vi "BK Precision 91xx (GPIB) Initialization VI.vi"(8 "error in (no error)":errorcluster, 10 "Custom XML":string, 11 "Device Item Ref in":T3 format="%.0x") -> (0 "error out":errorcluster, 3 "Device Item Ref out":T3 format="%.0x")   [LabVIEW 2009, in "BK Precision 91xx (GPIB) Custom Device.lvlib"]
uses:
  BK Precision 91xx (GPIB) Custom Device.lvlib
  <vilib>/NI VeriStand/Custom Device API/Custom Device Item Ref.ctl
  <vilib>/NI VeriStand/Custom Device API/Custom Device Channel.ctl
  <vilib>/NI VeriStand/Custom Device API/Custom Device Channel Type.ctl
  <vilib>/NI VeriStand/Custom Device API/Custom Device Timed Loop Priority.ctl
  <vilib>/NI VeriStand/Custom Device API/Custom Device Loop Type.ctl
  <vilib>/NI VeriStand/Custom Device API/Custom Device API.lvlib
panel:
  in  "Enable Channel":T1={"Type"=enum."Input", "Units"="", "Default Value"=0.0, "Faultable"=TRUE, "Scalable"=FALSE}
  in  "Output Channels":T1={"Type"=enum."Output", "Units"="", "Default Value"=0.0, "Faultable"=FALSE, "Scalable"=FALSE}
  in  "Input Channels":T1={"Type"=enum."Input", "Units"="Amps", "Default Value"=0.0, "Faultable"=TRUE, "Scalable"=TRUE}
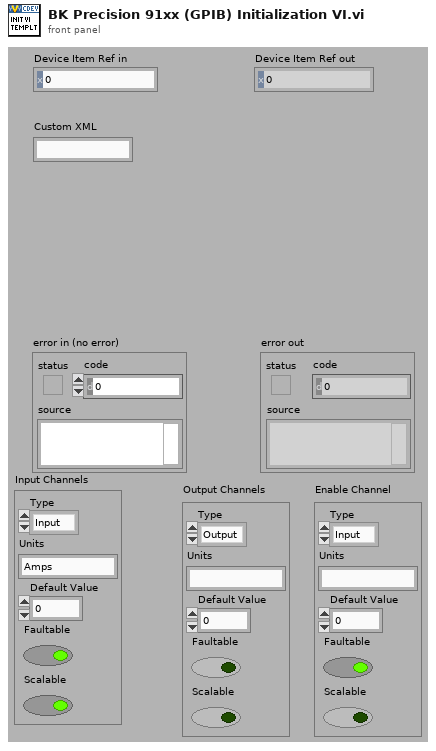
[diagram p1: front panel]
types:
  T1 = typedef "Custom Device API.lvlib/Custom Device Channel.ctl" = cluster{"Type":T2, "Units":string, "Default Value":dbl, "Faultable":bool, "Scalable":bool}
  T2 = typedef "Custom Device API.lvlib/Custom Device Channel Type.ctl" = enum16{"Input", "Output"}
  T3 = typedef "Custom Device API.lvlib/Custom Device Item Ref.ctl" = u64
  T4 = typedef "Custom Device API.lvlib/Custom Device Timed Loop Priority.ctl" = enum32{"Low", "Medium", "High"}
  T5 = typedef "Custom Device API.lvlib/Custom Device Loop Type.ctl" = enum32{"While Loop", "Timed Loop"}
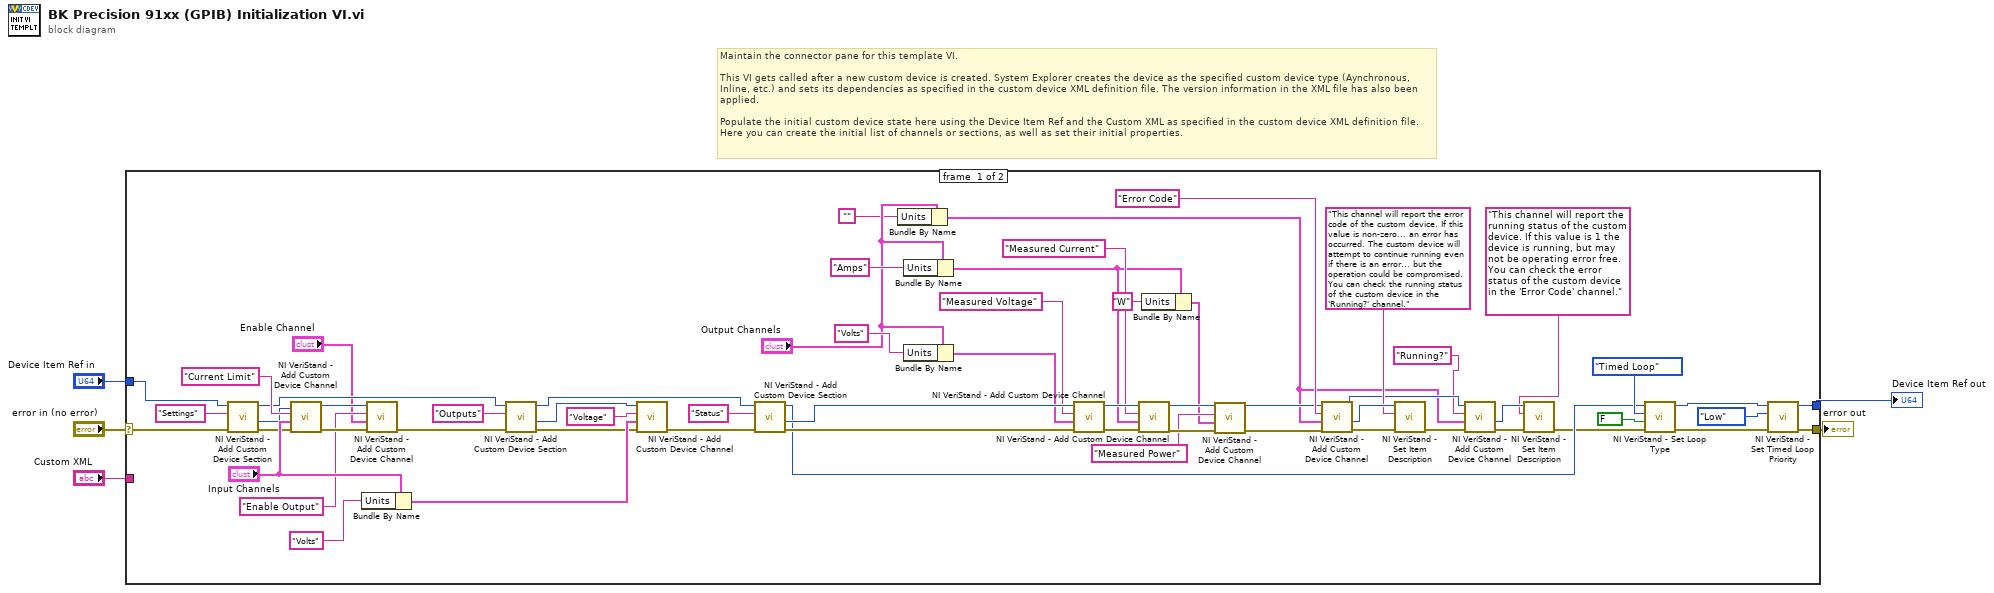
[diagram p0: block diagram]
diagram:
  # "Maintain the connector pane for this template VI.\n\nThis VI gets called after a new custom device is created. System Explorer creates the device as the specified custom device type (Aynchronous, Inline, etc.) and sets its dependencies as specified in the custom device XML definition file. The version information in the XML file has also been applied.\n\nPopulate the initial custom device state here using the Device Item Ref and the Custom XML as specified in the custom device XML definition file. Here you can create the initial list of channels or sections, as well as set their initial properties."
  n1 = case shown="No Error" "error in (no error)" {
    selector: "error in (no error)" -> [w40 w68]
    tunnel: [w48 w68] -> w5
    tunnel: [w45 w67] -> w3
    tunnel: "Device Item Ref in" -> [w41 w67]
    tunnel: "Custom XML" -> [_ _]
    frame #0 {
      n2 = call <vilib>:"NI VeriStand - Add Custom Device Section.vi"("error in (no error)"=w40, "Section Name"="Settings", "Parent Ref in"=w41) -> ("error out"=w36:errorcluster, "Section Ptr"=w39:T3, "Parent Ref out"=w32:T3)  [unwired: 6 in]
      n3 = call <vilib>:"NI VeriStand - Add Custom Device Channel.vi"("error in (no error)"=w36, "Channel"="Input Channels", "Channel Name"="Current Limit", "Parent Ref in"=w39) -> ("error out"=w33:errorcluster, "Parent Ref out"=w31:T3)  [unwired: 5 in, 1 out]
      n4 = Bundle By Name(cluster="Input Channels", "Units"="Volts") -> (w58:T1)
      n5 = call <vilib>:"NI VeriStand - Add Custom Device Channel.vi"("error in (no error)"=w33, "Channel"="Enable Channel", "Channel Name"="Enable Output", "Parent Ref in"=w31) -> ("error out"=w34:errorcluster)  [unwired: 5 in, 2 out]
      n6 = call <vilib>:"NI VeriStand - Add Custom Device Section.vi"("error in (no error)"=w34, "Section Name"="Outputs", "Parent Ref in"=w32) -> ("error out"=w35:errorcluster, "Section Ptr"=w38:T3, "Parent Ref out"=w62:T3)  [unwired: 6 in]
      n7 = call <vilib>:"NI VeriStand - Add Custom Device Channel.vi"("error in (no error)"=w35, "Channel"=w58, "Channel Name"="Voltage", "Parent Ref in"=w38) -> ("error out"=w63:errorcluster)  [unwired: 5 in, 2 out]
      n8 = call <vilib>:"NI VeriStand - Add Custom Device Section.vi"("error in (no error)"=w63, "Section Name"="Status", "Parent Ref in"=w62) -> ("error out"=w57:errorcluster, "Section Ptr"=w56:T3, "Parent Ref out"=w22:T3)  [unwired: 6 in]
      n9 = Bundle By Name(cluster="Output Channels", "Units"="") -> (w7:T1)
      n10 = Bundle By Name(cluster="Output Channels", "Units"="Amps") -> (w18:T1)
      n11 = Bundle By Name(cluster="Output Channels", "Units"="Volts") -> (w50:T1)
      n12 = call <vilib>:"NI VeriStand - Add Custom Device Channel.vi"("error in (no error)"=w57, "Channel"=w50, "Channel Name"="Measured Voltage", "Parent Ref in"=w56) -> ("error out"=w53:errorcluster, "Parent Ref out"=w54:T3)  [unwired: 5 in, 1 out]
      n13 = call <vilib>:"NI VeriStand - Add Custom Device Channel.vi"("error in (no error)"=w53, "Channel"=w18, "Channel Name"="Measured Current", "Parent Ref in"=w54) -> ("error out"=w21:errorcluster, "Parent Ref out"=w20:T3)  [unwired: 5 in, 1 out]
      n14 = Bundle By Name(cluster=w18, "Units"="W") -> (w16:T1)
      n15 = call <vilib>:"NI VeriStand - Add Custom Device Channel.vi"("error in (no error)"=w21, "Channel"=w16, "Channel Name"="Measured Power", "Parent Ref in"=w20) -> ("error out"=w15:errorcluster, "Parent Ref out"=w14:T3)  [unwired: 5 in, 1 out]
      n16 = call <vilib>:"NI VeriStand - Add Custom Device Channel.vi"("error in (no error)"=w15, "Channel"=w7, "Channel Name"="Error Code", "Parent Ref in"=w14) -> ("error out"=w25:errorcluster, "Channel Ref"=w24:T3, "Parent Ref out"=w12:T3)  [unwired: 5 in]
      n17 = call <vilib>:"NI VeriStand - Set Item Description.vi"("error in (no error)"=w25, "Description"="This channel will report the error code of the custom device. If this value is non-zero... an error has occurred. The custom device will attempt to continue running even if there is an error... but the operation could be compromised. You can check the running status of the custom device in the 'Running?' channel.", "Item Ref in"=w24) -> ("error out"=w13:errorcluster)  [unwired: 6 in, 2 out]
      n18 = call <vilib>:"NI VeriStand - Add Custom Device Channel.vi"("error in (no error)"=w13, "Channel"=w7, "Channel Name"="Running?", "Parent Ref in"=w12) -> ("error out"=w11:errorcluster, "Channel Ref"=w9:T3)  [unwired: 5 in, 1 out]
      n19 = call <vilib>:"NI VeriStand - Set Item Description.vi"("error in (no error)"=w11, "Description"="This channel will report the running status of the custom device. If this value is 1 the device is running, but may not be operating error free.  You can check the error status of the custom device in the 'Error Code' channel.", "Item Ref in"=w9) -> ("error out"=w10:errorcluster)  [unwired: 6 in, 2 out]
      n20 = call <vilib>:"NI VeriStand - Set Loop Type.vi"("error in (no error)"=w10, "Use Device Clock (Timed Loops only)"=FALSE, "Loop type"=Custom_Device_Loop_Type."Timed Loop", "Device Ref in"=w22) -> ("error out"=w47:errorcluster, "Device Ref out"=w46:T3)  [unwired: 6 in]
      n21 = call <vilib>:"NI VeriStand - Set Timed Loop Priority.vi"("error in (no error)"=w47, "Priority"=Custom_Device_Timed_Loop_Priority."Low", "Device Ref in"=w46) -> ("error out"=w48:errorcluster, "Device Ref out"=w45:T3)  [unwired: 7 in]
    }
    frame #1 {
    }
  }
  "error out" <- w5
  "Device Item Ref out" <- w3
